vi "lev-mar template.vi"   [LabVIEW 2010]
uses:
  <vilib>/gmath/NumericalOptimization/LM model function reference.ctl
  <vilib>/gmath/NI_Gmath.lvlib
  <vilib>/gmath/NumericalOptimization/Nonlinear Curve Fit LM.vi
  <vilib>/gmath/NumericalOptimization/Nonlinear Curve Fit LM formula string.vi
types:
  T1 = cluster{"model":string, "Parameters":string[], "x":string}
  T2 = typedef "NI_Gmath.lvlib/LM model function reference.ctl" = refnum<vi>
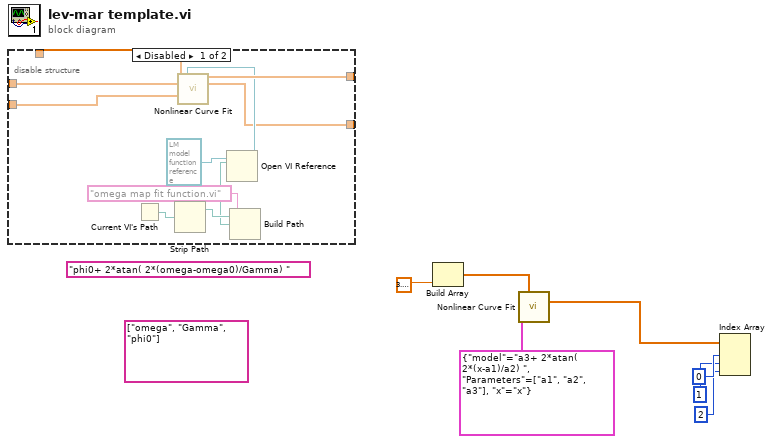
[diagram p0: block diagram]
diagram:
  (unwired) string[] ["omega", "Gamma", "phi0"] ("Parameters")
  (unwired) "phi0+ 2*atan( 2*(omega-omega0)/Gamma) " ("model")
  n1 = disable-structure shown="Disabled" {
    disable-tunnel: _ -> [w23 _]
    disable-tunnel: [w22 _] -> _
    disable-tunnel: _ -> [w15 _]
    disable-tunnel: _ -> [w14 _]
    disable-tunnel: [w13 _] -> _
    frame Disabled {
      n2 = Current VI's Path() -> (path=w20:path)
      n3 = Strip Path(path=w20) -> (stripped path=w19:path)  [unwired: 1 out]
      n4 = Build Path(base path=w19, name or relative path="omega map fit function.vi" ("f(x,a) VI name Complex")) -> (appended path=w17:path)
      n5 = Open VI Reference(type specifier VI Refnum (for type only)=T2 refnum ("f(x,a)"), vi path=w17) -> (vi reference=w16:T2)  [unwired: 1 in, 4 out]
      n6 = call-poly <vilib>:"Nonlinear Curve Fit.vi"("Y"=w14, "f(x,a)"=w16, "X"=w15, "initial parameters"=w23) -> ("best nonlinear fit"=w22:dbl[], "best fit parameters"=w13:dbl[])  [unwired: 6 in, 4 out]
    }
    frame Enabled {
    }
  }
  n7 = Build Array(3.141592653589793) -> (w10:dbl[], w6:dbl, w7:dbl)
  n8 = call-poly <vilib>:"Nonlinear Curve Fit.vi"("initial parameters"=w10, "model description"=T1 {"model"="a3+ 2*atan( 2*(x-a1)/a2) ", "Parameters"=["a1", "a2", "a3"], "x"="x"}) -> ("Y"=w8:dbl[], "best nonlinear fit"=w9:dbl[], "X"=w12:dbl[], "best fit parameters"=w5:dbl[])  [unwired: 7 in, 3 out]
  n9 = Index Array(array=w5, index #1=0, index #2=1, index #3=2) -> ()  [unwired: 3 out]
